vi "IniHSSpeeds.vi"(4 "error out 2":errorcluster, 5 "DLL error code":u32, 6 "number":i32, 7 "Boolean":bool) -> (0 "error out":errorcluster, 2 "to shell":string caption="Result", 3 "Numeric":i32)   [LabVIEW 2011]
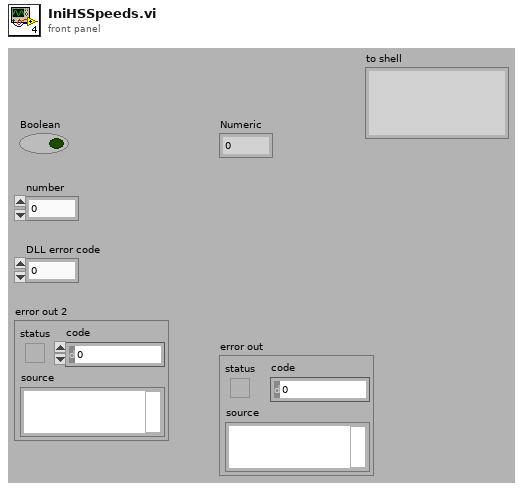
[diagram p1: front panel]
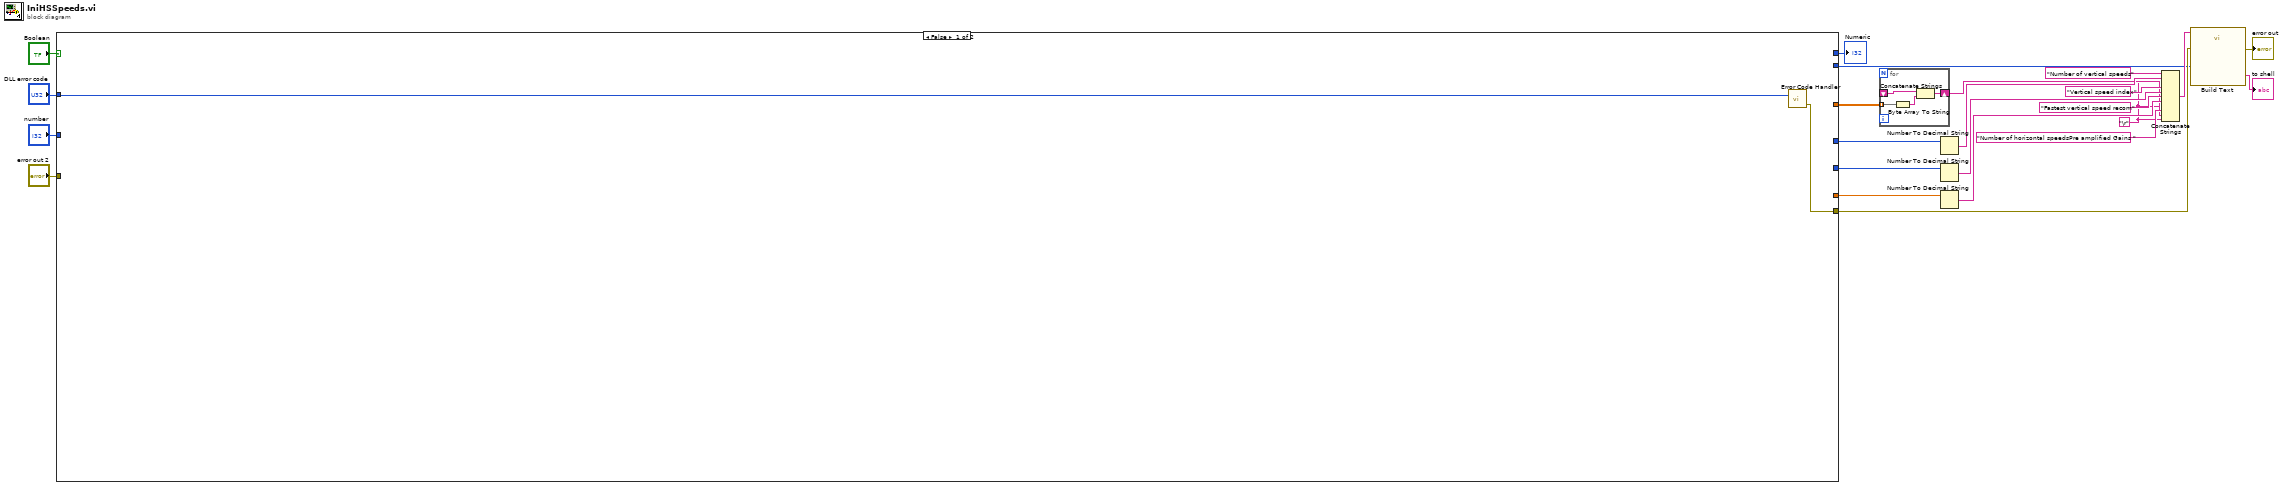
[diagram p0: block diagram]
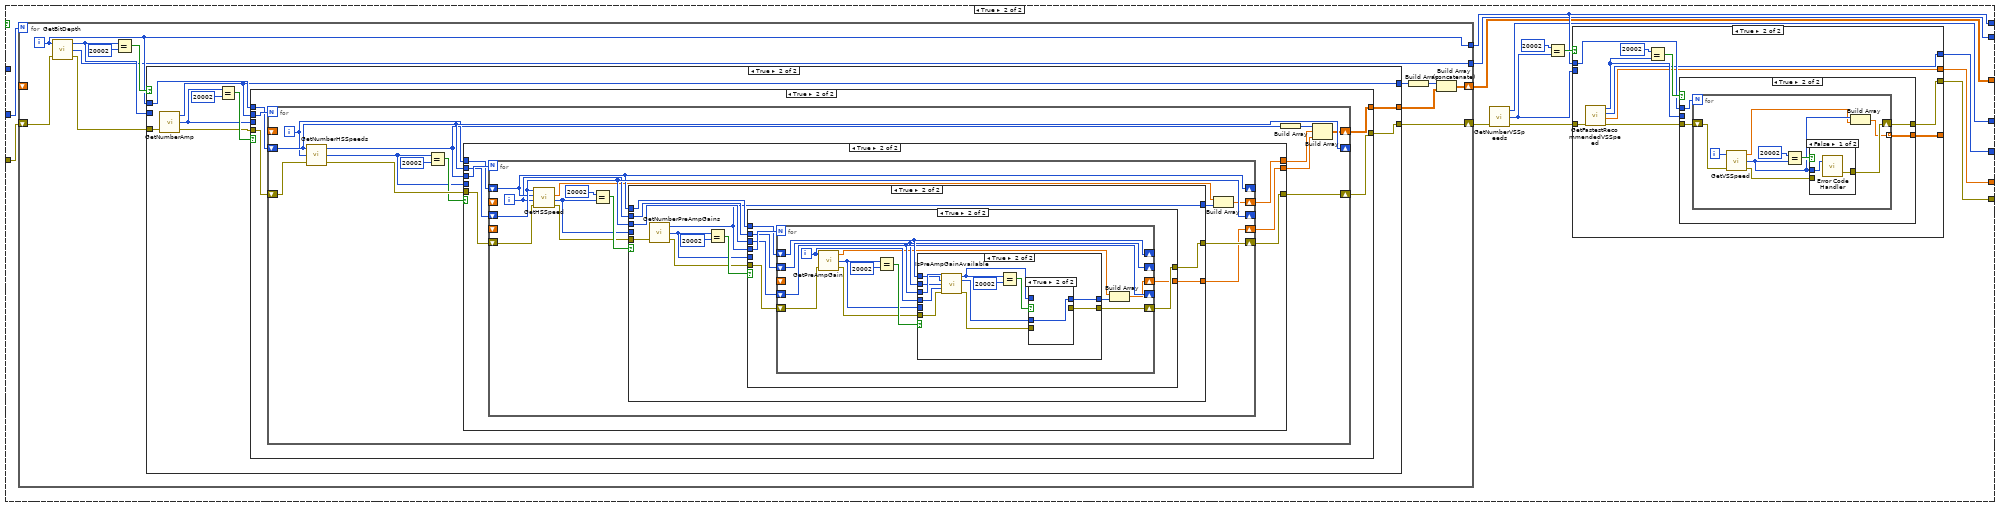
[diagram p2: hidden frame]
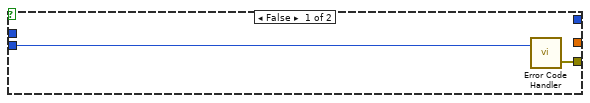
[diagram p3: hidden frame]
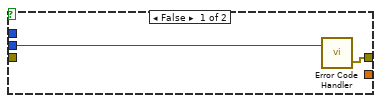
[diagram p4: hidden frame]
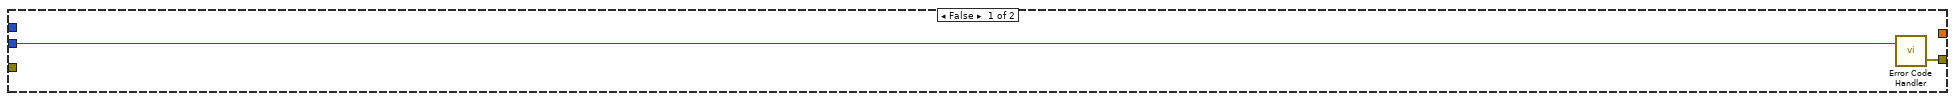
[diagram p6: hidden frame]
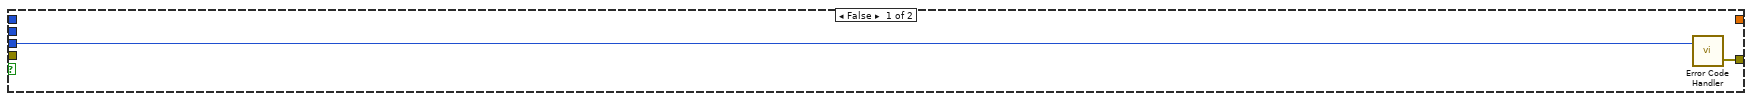
[diagram p7: hidden frame]
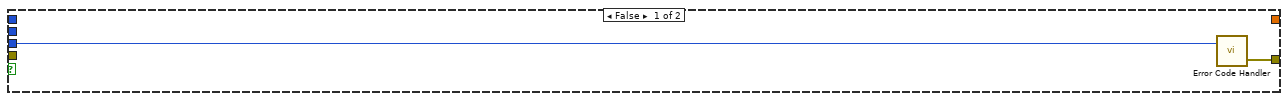
[diagram p8: hidden frame]
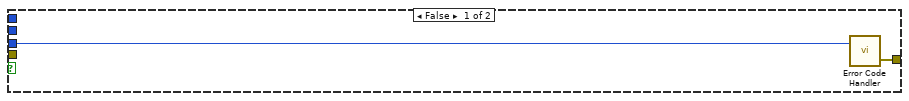
[diagram p9: hidden frame]
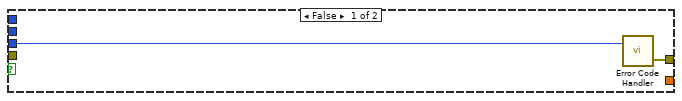
[diagram p10: hidden frame]
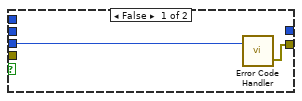
[diagram p11: hidden frame]
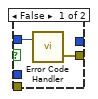
[diagram p12: hidden frame]
diagram:
  w2 = "\r"
  n1 = case shown="False" "Boolean" {
    tunnel: "number" -> [_ w33]
    tunnel: "DLL error code" -> [w25 _]
    tunnel: [w24 w34] -> w8
    tunnel: "error out 2" -> [_ w39]
    tunnel: [_ w32] -> w22
    tunnel: [_ w30] -> w5
    tunnel: [_ w29] -> w18
    tunnel: [_ w28] -> w17
    tunnel: [_ w27] -> w16
    tunnel: [_ w26] -> w6
    frame False {
      n2 = call "Error Code Handler.vi"("DLL error code"=w25) -> ("error out"=w24:errorcluster)  [unwired: 1 in, 1 out]
    }
    frame True {
      n3 = for {
        N: w33 -> [_]
        shift-right: [w77] -> w35
        shift-left: w39 -> [w81]
        tunnel: [w75] -> w32
        shift-right: [w73] -> w30
        shift-left: _ -> [_]
        tunnel: [w72] -> w26
        i -> [w75]
        n4 = call "GetBitDepth.vi"("error in (no error)"=w81, "channel"=w75) -> ("error out"=w78:errorcluster, "depth"=w72:i32, "DLL error code"=w76:u32)  [unwired: 1 in]
        n5 = Equal?(x=w76, y=u32 20002) -> (x = y?=w79:bool)
        n6 = case shown="True" w79 {
          tunnel: w76 -> [w83 _]
          tunnel: w78 -> [_ w92]
          tunnel: [w82 w88] -> w77
          tunnel: w75 -> [_ w87]
          tunnel: [_ w85] -> w71
          tunnel: [_ w84] -> w74
          frame False {
            n7 = call "Error Code Handler.vi"("DLL error code"=w83) -> ("error out"=w82:errorcluster)  [unwired: 1 in, 1 out]
          }
          frame True {
            n8 = call "GetNumberAmp.vi"("error in (no error)"=w92) -> ("error out"=w89:errorcluster, "DLL error code"=w86:u32, "number"=w85:i32)  [unwired: 2 in]
            n9 = Equal?(x=w86, y=u32 20002) -> (x = y?=w90:bool)
            n10 = case shown="True" w90 {
              tunnel: w89 -> [_ w98]
              tunnel: [w94 w97] -> w88
              tunnel: w86 -> [w93 _]
              tunnel: w85 -> [_ w99]
              tunnel: w87 -> [_ w96]
              tunnel: [_ w95] -> w84
              frame False {
                n11 = call "Error Code Handler.vi"("DLL error code"=w93) -> ("error out"=w94:errorcluster)  [unwired: 1 in, 1 out]
              }
              frame True {
                n12 = for {
                  N: w99 -> [_]
                  shift-right: [w110] -> w97
                  shift-left: w98 -> [w112]
                  shift-right: [w107] -> _
                  shift-left: w96 -> [w107]
                  shift-right: [w100] -> w95
                  shift-left: _ -> [_]
                  i -> [w106]
                  n13 = call "GetNumberHSSpeeds.vi"("error in (no error)"=w112, "type"=w106, "channel"=w107) -> ("error out"=w111:errorcluster, "DLL error code"=w104:u32, "number"=w105:i32)
                  n14 = Equal?(x=w104, y=u32 20002) -> (x = y?=w108:bool)
                  n15 = case shown="True" w108 {
                    tunnel: w111 -> [_ w121]
                    tunnel: [w114 w120] -> w110
                    tunnel: w105 -> [_ w119]
                    tunnel: w104 -> [w113 _]
                    tunnel: w107 -> [_ w118]
                    tunnel: w106 -> [_ w117]
                    tunnel: [_ w116] -> w103
                    tunnel: [_ w115] -> w102
                    frame False {
                      n16 = call "Error Code Handler.vi"("DLL error code"=w113) -> ("error out"=w114:errorcluster)  [unwired: 1 in, 1 out]
                    }
                    frame True {
                      n17 = for {
                        N: w119 -> [_]
                        shift-right: [w130] -> w120
                        shift-left: w121 -> [w134]
                        shift-right: [w129] -> _
                        shift-left: w118 -> [w129]
                        shift-right: [w128] -> _
                        shift-left: w117 -> [w128]
                        shift-right: [w123] -> w116
                        shift-left: _ -> [_]
                        shift-right: [w122] -> w115
                        shift-left: _ -> [_]
                        i -> [w127]
                        n18 = call "GetHSSpeed.vi"("error in (no error)"=w134, "index"=w127, "type"=w128, "channel"=w129) -> ("error out"=w131:errorcluster, "DLL error code"=w125:u32, "speed"=w126:sgl)  [unwired: 1 in]
                        n19 = Equal?(x=u32 20002 ("y"), y=w125) -> (x = y?=w133:bool)
                        n20 = case shown="True" w133 {
                          tunnel: w131 -> [_ w147]
                          tunnel: [w136 w143] -> w130
                          tunnel: w129 -> [_ w142]
                          tunnel: w125 -> [w135 _]
                          tunnel: w128 -> [_ w141]
                          tunnel: w127 -> [_ w140]
                          tunnel: [_ w139] -> w124
                          tunnel: [_ w137] -> w122
                          frame False {
                            n21 = call "Error Code Handler.vi"("DLL error code"=w135) -> ("error out"=w136:errorcluster)  [unwired: 1 in, 1 out]
                          }
                          frame True {
                            n22 = call "GetNumberPreAmpGains.vi"("error in (no error)"=w147) -> ("error out"=w144:errorcluster, "DLL error code"=w138:u32, "number"=w139:i32)  [unwired: 2 in]
                            n23 = Equal?(x=w138, y=u32 20002) -> (x = y?=w146:bool)
                            n24 = case shown="True" w146 {
                              tunnel: w139 -> [_ w156]
                              tunnel: w144 -> [_ w155]
                              tunnel: [w149 w154] -> w143
                              tunnel: w142 -> [_ w153]
                              tunnel: w138 -> [w148 _]
                              tunnel: w141 -> [_ w152]
                              tunnel: w140 -> [_ w151]
                              tunnel: [_ w150] -> w137
                              frame False {
                                n25 = call "Error Code Handler.vi"("DLL error code"=w148) -> ("error out"=w149:errorcluster)  [unwired: 1 in, 1 out]
                              }
                              frame True {
                                n26 = for {
                                N: w156 -> [_]
                                shift-right: [w165] -> w154
                                shift-left: w155 -> [w169]
                                shift-right: [w163] -> _
                                shift-left: w153 -> [w163]
                                shift-right: [w164] -> _
                                shift-left: w152 -> [w164]
                                shift-right: [w162] -> _
                                shift-left: w151 -> [w162]
                                shift-right: [w157] -> w150
                                shift-left: _ -> [_]
                                i -> [w161]
                                n27 = call "GetPreAmpGain.vi"("error in (no error)"=w169, "index"=w161) -> ("error out"=w166:errorcluster, "DLL error code"=w159:u32, "gain"=w160:sgl)  [unwired: 1 in]
                                n28 = Equal?(x=w159, y=u32 20002) -> (x = y?=w167:bool)
                                n29 = case shown="True" w167 {
                                tunnel: w166 -> [_ w183]
                                tunnel: [w171 w175] -> w165
                                tunnel: w163 -> [_ w182]
                                tunnel: w159 -> [w170 _]
                                tunnel: w164 -> [_ w181]
                                tunnel: w162 -> [_ w180]
                                tunnel: w161 -> [_ w179]
                                tunnel: [_ w173] -> w158
                                frame False {
                                n30 = call "Error Code Handler.vi"("DLL error code"=w170) -> ("error out"=w171:errorcluster)  [unwired: 1 in, 1 out]
                                }
                                frame True {
                                n31 = call "IsPreAmpGainAvailable.vi"("channel"=w182, "amplifier"=w181, "index"=w180, "pa"=w179, "error in (no error)"=w183) -> ("DLL error code"=w172:u32, "status"=w174:i32, "error out"=w176:errorcluster)  [unwired: 8 in]
                                n32 = Equal?(x=w172, y=u32 20002) -> (x = y?=w177:bool)
                                n33 = case shown="True" w177 {
                                tunnel: w176 -> [_ _]
                                tunnel: [w185 _] -> w175
                                tunnel: w172 -> [w184 _]
                                tunnel: w174 -> [_ w186]
                                tunnel: [_ w186] -> w173
                                frame False {
                                n34 = call "Error Code Handler.vi"("DLL error code"=w184) -> ("error out"=w185:errorcluster)  [unwired: 1 in, 1 out]
                                }
                                frame True {
                                }
                                }
                                }
                                }
                                n35 = Build Array(w160, w158) -> (w157:sgl[])
                                }
                              }
                            }
                          }
                        }
                        n36 = Build Array(w126, w124) -> (w123:sgl[])
                      }
                    }
                  }
                  n37 = Build Array(w105) -> (w101:i32[])
                  n38 = Build Array(w101, w103, w102) -> (w100:sgl[][])
                }
              }
            }
          }
        }
        n39 = Build Array(w71) -> (w70:i32[])
        n40 = Build Array (concatenate)(w70, w74) -> (w73:sgl[][])
      }
      n41 = call "GetNumberVSSpeeds.vi"("error in (no error)"=w35) -> ("error out"=w36:errorcluster, "DLL error code"=w31:u32, "number"=w29:i32)  [unwired: 2 in]
      n42 = Equal?(x=u32 20002, y=w31) -> (x = y?=w37:bool)
      n43 = case shown="True" w37 {
        tunnel: w31 -> [w41 _]
        tunnel: [w40 w48] -> w34
        tunnel: w36 -> [_ w51]
        tunnel: w32 -> [_ w47]
        tunnel: [_ w44] -> w28
        tunnel: [_ w43] -> w27
        tunnel: [_ w42] -> _
        frame False {
          n44 = call "Error Code Handler.vi"("DLL error code"=w41) -> ("error out"=w40:errorcluster)  [unwired: 1 in, 1 out]
        }
        frame True {
          n45 = call "GetFastestRecommendedVSSpeed.vi"("error in (no error)"=w51) -> ("error out"=w46:errorcluster, "speed"=w43:sgl, "index"=w44:u32, "DLL error code"=w45:u32)  [unwired: 3 in]
          n46 = Equal?(x=u32 20002, y=w45) -> (x = y?=w49:bool)
          n47 = case shown="True" w49 {
            tunnel: [w53 w55] -> w48
            tunnel: w45 -> [w52 _]
            tunnel: w47 -> [_ w57]
            tunnel: w46 -> [_ w56]
            tunnel: [_ w54] -> w42
            frame False {
              n48 = call "Error Code Handler.vi"("DLL error code"=w52) -> ("error out"=w53:errorcluster)  [unwired: 1 in, 1 out]
            }
            frame True {
              n49 = for {
                N: w57 -> [_]
                shift-right: [w62] -> w55
                shift-left: w56 -> [w66]
                tunnel: [w58] -> w54 mode=indexing
                i -> [w61]
                n50 = call "GetVSSpeed.vi"("error in (no error)"=w66, "index"=w61) -> ("error out"=w63:errorcluster, "DLL error code"=w60:u32, "speed"=w59:sgl)  [unwired: 1 in]
                n51 = Equal?(x=u32 20002, y=w60) -> (x = y?=w64:bool)
                n52 = case shown="False" w64 {
                  tunnel: w63 -> [_ w69]
                  tunnel: [w68 w69] -> w62
                  tunnel: w60 -> [w67 _]
                  frame False {
                    n53 = call "Error Code Handler.vi"("DLL error code"=w67) -> ("error out"=w68:errorcluster)  [unwired: 1 in, 1 out]
                  }
                  frame True {
                  }
                }
                n54 = Build Array(w60, w59) -> (w58:sgl[])
              }
            }
          }
        }
      }
    }
  }
  "Numeric" <- w22
  n55 = for {
    tunnel: w5 -> [w190] mode=indexing
    shift-right: [w187] -> w3
    shift-left: _ -> [w188]
    n56 = Byte Array To String(unsigned byte array=w190) -> (string=w189:string)
    n57 = Concatenate Strings(w188, w189) -> (w187:string)
  }
  n58 = Number To Decimal String(number=w18) -> (decimal integer string=w14:string)  [unwired: 1 in]
  n59 = Number To Decimal String(number=w17) -> (decimal integer string=w12:string)  [unwired: 1 in]
  n60 = Number To Decimal String(number=w16) -> (decimal integer string=w10:string)  [unwired: 1 in]
  n61 = Concatenate Strings("Number of vertical speeds" ("string"), w14, w2, "Vertical speed index" ("string"), w12, "Fastest vertical speed recom" ("string"), w10, w2, "Number of horizontal speedsPre amplified Gains " ("string"), w3, w2) -> (w9:string)
  n62 = call "Build Text"("Beginning Text"=w9, "bit"=w6, "error in (no error)"=w8) -> ("Result"=→"to shell":string, "error out"=→"error out":errorcluster)  [unwired: 11 in]
